vi "DOWNLOAD USER PHOTO.vi"(11 "BYU ID #":string) -> (3 "Image String Out":string)   [LabVIEW 2019]
uses:
  <vilib>/addons/database/Connection.llb/DB Tools Open Connec (String).vi
  <vilib>/regexp/Match Regular Expression.xnode
  <vilib>/addons/database/NI_Database_API.lvlib
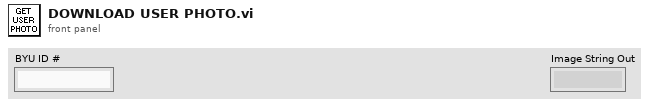
[diagram p1: front panel]
types:
  T1 = typedef "Image Type" = u32
  T2 = typedef "IMAQ Image.ctl" = refnum<image>
  T3 = typedef "NI_Database_API.lvlib/Conn ObjectReference.ctl" = refnum<k1>
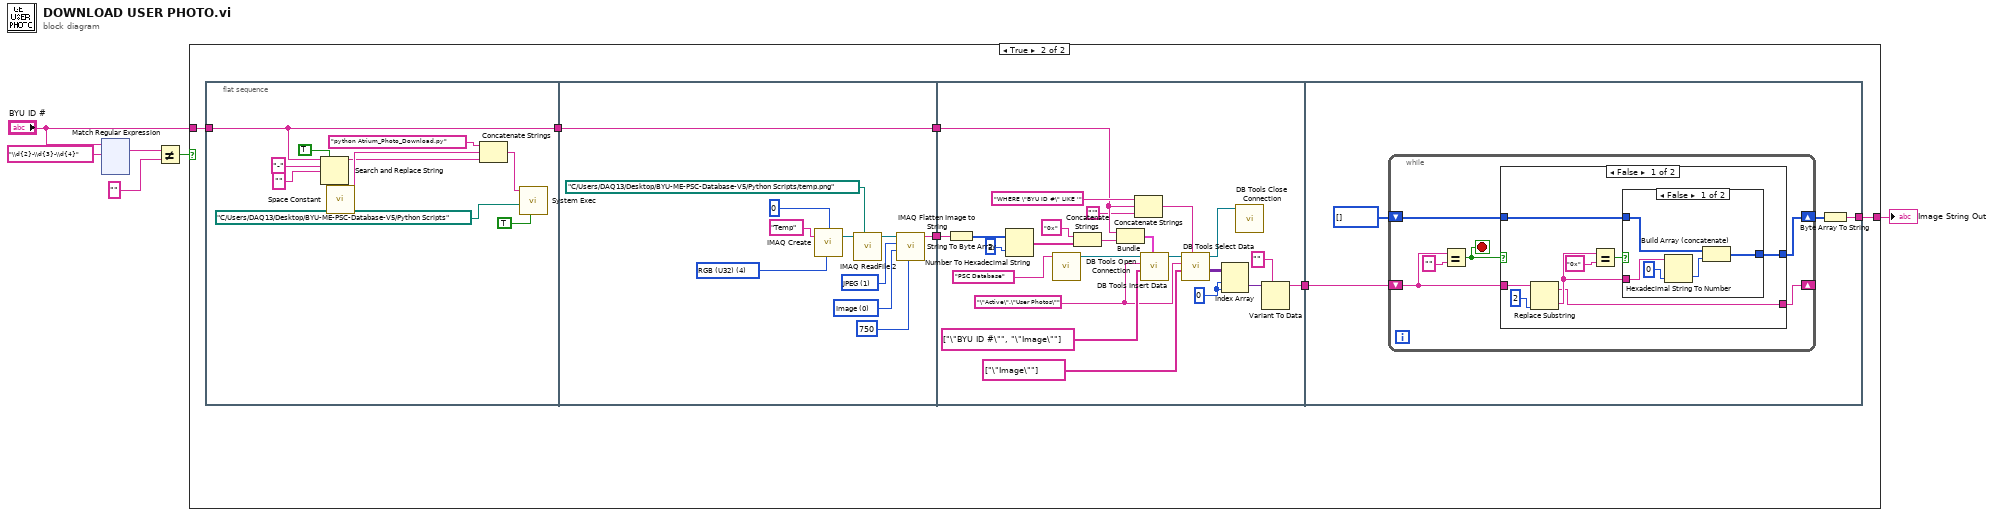
[diagram p0: block diagram]
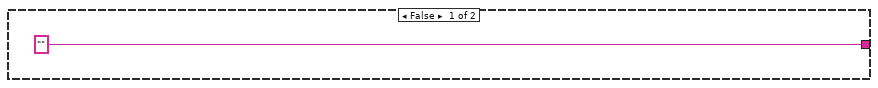
[diagram p2: hidden frame]
diagram:
  n1 = xnode "Match Regular Expression"("input string"="BYU ID #", "regular expression"="\\d{2}-\\d{3}-\\d{4}") -> ("whole match"=w4:string)  [unwired: 4 in, 4 out]
  n2 = Not Equal?(x=w4, y="") -> (x != y?=w1:bool)
  n3 = case shown="True" w1 {
    tunnel: "BYU ID #" -> [_ w9]
    tunnel: ["" ("string") w8] -> w2
    frame False {
    }
    frame True {
      n4 = flat-sequence {
        tunnel: w9 -> [w23]
        tunnel: [w23] -> w13
        tunnel: [w28] -> w12
        tunnel: [w24] -> w11
        tunnel: w13 -> [w24]
        tunnel: w12 -> [w45]
        tunnel: [w41] -> w10
        tunnel: w11 -> [w37]
        tunnel: w10 -> [w61]
        tunnel: [w58] -> w8
        frame #0 {
          n5 = Search and Replace String(replace all?=TRUE ("replace all? (F)"), input string=w23, search string="-", replace string="" ("replace string (\"\")")) -> (result string=w17:string)  [unwired: 4 in, 3 out]
          n6 = call <vilib>:"Space Constant.vi"() -> ("String"=w18:string)
          n7 = Concatenate Strings("python Atrium_Photo_Download.py" ("command line"), w18, w17) -> (w16:string)
          n8 = call <vilib>:"System Exec.vi"("run minimized? (F)"=TRUE, "working directory"=path "C:/Users/DAQ13/Desktop/BYU-ME-PSC-Database-V5/Python Scripts" ("File Path"), "command line"=w16) -> ()  [unwired: 5 in, 4 out]
        }
        frame #1 {
          w26 = 0 items=["Image", "Image and Vision Info", "Reference to Image"] ("Type of Flatten (Image and Vision Info)")
          w27 = 1 items=["None", "JPEG", "PACKED BINARY"] ("Compression (None)")
          w32 = T1 4 items=["Grayscale (U8)", "Grayscale (I16)", "Grayscale (SGL)", "Complex (CSG)", "RGB (U32)", "HSL (U32)", "RGB (U64)", "Grayscale (U16)"] ("Image Type")
          n9 = call "IMAQ Create"("Border Size"=0, "Image Name"="Temp", "Image Type"=w32) -> ("New Image"=w34:T2)  [unwired: 2 in, 1 out]
          n10 = call "IMAQ ReadFile 2"("File Path"=path "C:/Users/DAQ13/Desktop/BYU-ME-PSC-Database-V5/Python Scripts/temp.png", "Image"=w34) -> ("Image Out"=w29:T2)  [unwired: 5 in, 4 out]
          n11 = call "IMAQ Flatten Image to String"("Quality (750)"=750, "Type of Flatten (Image and Vision Info)"=w26, "Compression (None)"=w27, "Image"=w29) -> ("Data String"=w28:string)  [unwired: 6 in, 1 out]
        }
        frame #2 {
          w51 = 0 ("disabled index (col)")
          w47 = "\"Active\".\"User Photos\"" ("table")
          n12 = String To Byte Array(string=w45) -> (unsigned byte array=w40:u8[])
          n13 = Number To Hexadecimal String(1:i16 2 ("width (-)"), 2:w40) -> (0:w43:string[])
          n14 = call-poly <vilib>:"DB Tools Open Connection.vi"("connection information"="PSC Database") -> ("connection reference"=w56:T3)  [unwired: 7 in, 1 out]
          n15 = Concatenate Strings("0x" ("string"), w43) -> (w42:string)
          n16 = Bundle("BYU ID #"=w37, w42) -> (w39:cluster{"BYU ID #":string, string})  [unwired: 1 in]
          n17 = Concatenate Strings("WHERE \"BYU ID #\" LIKE '" ("SQL query"), w37, "'" ("element")) -> (w35:string)
          n18 = call <vilib>:"DB Tools Insert Data.vi"("data"=w39, "columns"=string[] ["\"BYU ID #\"", "\"Image\""], "table"=w47, "connection reference"=w56) -> ("connection reference out"=w55:T3)  [unwired: 6 in, 1 out]
          n19 = call <vilib>:"DB Tools Select Data.vi"("condition"=w35, "columns"=string[] ["\"Image\""], "table"=w47, "connection reference"=w55) -> ("data"=w52:variant[][], "connection reference out"=w53:T3)  [unwired: 2 in, 1 out]
          n20 = Index Array(array=w52, index (row)=w51, index (col)=w51) -> (element=w49:variant)
          n21 = call <vilib>:"DB Tools Close Connection.vi"("connection reference"=w53) -> ()  [unwired: 6 in, 1 out]
          n22 = Variant To Data(type="" ("concatenated string"), Variant=w49) -> (data=w41:string)  [unwired: 1 in, 1 out]
        }
        frame #3 {
          n23 = while {
            shift-right: [w62] -> _
            shift-left: w61 -> [w65]
            shift-right: [w66] -> w59
            shift-left: u8[] [] ("unsigned byte array") -> [w67]
            stop <- w63 stop-if-true
            n24 = Equal?(x=w65, y="") -> (x = y?=w63:bool)
            n25 = case shown="False" w63 {
              tunnel: w67 -> [w72 w82]
              tunnel: [w71 w82] -> w66
              tunnel: [w68 w83] -> w62
              tunnel: w65 -> [w69 w83]
              frame False {
                n26 = Replace Substring(2:2 ("length (len. of substring)"), 5:w69) -> (0:w70:string, 1:w68:string)  [unwired: 2 in]
                n27 = Equal?(x=w70, y="0x") -> (x = y?=w73:bool)
                n28 = case shown="False" w73 {
                  tunnel: w72 -> [w78 w81]
                  tunnel: [w76 w81] -> w71
                  tunnel: w70 -> [w80 _]
                  frame False {
                    n29 = Hexadecimal String To Number(string=w80, default (0uL)=u8 0) -> (number=w77:u8)  [unwired: 1 in, 1 out]
                    n30 = Build Array (concatenate)(w78, w77) -> (w76:u8[])
                  }
                  frame True {
                  }
                }
              }
              frame True {
              }
            }
          }
          n31 = Byte Array To String(unsigned byte array=w59) -> (string=w58:string)
        }
      }
    }
  }
  "Image String Out" <- w2
